vi "Lab Panel V6.00.vi"() -> ()   [LabVIEW 2017] (continued)
              tunnel: w5250 -> [w5255 w5288]
              tunnel: w5249 -> [w5254 w5287]
              tunnel: w5248 -> [w5253 _]
              tunnel: w5237 -> [_ w5286]
              tunnel: w5247 -> [_ w5285]
              tunnel: w5246 -> [_ w5284]
              tunnel: w5245 -> [_ w5283]
              tunnel: w5244 -> [_ w5282]
              tunnel: w5243 -> [_ w5281]
              tunnel: w5242 -> [_ w5280]
              tunnel: w5241 -> [_ w5279]
              tunnel: w5240 -> [_ w5278]
              tunnel: w5239 -> [_ w5277]
              tunnel: w5238 -> [_ w5276]
              tunnel: "TO (string):" -> [w5252 _]
              frame #0 {
                # "mail test"
                n2915 = case shown="True" w5253 {
                  tunnel: w5256 -> [_ w5260]
                  tunnel: w5252 -> [_ w5259]
                  tunnel: w5255 -> [_ w5258]
                  tunnel: w5254 -> [_ w5257]
                  frame False {
                  }
                  frame True {
                    n2916 = stacked-sequence {
                      seq-local: [_ _ w5270 _] -> [_ _ _ w5271]
                      tunnel: w5260 -> [w5263 _ _ w5275]
                      tunnel: w5259 -> [_ _ w5268 _]
                      tunnel: w5258 -> [_ _ w5266 _]
                      tunnel: w5257 -> [_ _ w5267 _]
                      frame #0 {
                        n2917 = Bundle(cluster=w5263, "TEST MAIL STATUS"="TEST START") -> (w5261:T8)  [unwired: 6 in]
                        n2918 = local write "MAIL SETTINGS"(w5261) -> ()
                      }
                      frame #1 {
                        n2919 = Wait (ms)(milliseconds to wait=500) -> ()  [unwired: 1 out]
                      }
                      frame #2 {
                        n2920 = call "sub vi - send mail v5.vi"("TO:"=w5268, "subject"="MAIL TEST FROM LAB PANEL", "from"=w5267, "out going server"=w5266, "message"="TEST MESSAGE") -> ("error out"=w5270:errorcluster)  [unwired: 10 in]
                      }
                      frame #3 {
                        n2921 = Bundle(cluster=w5275, "TEST MAIL"=FALSE, "TEST MAIL STATUS"="TEST END", "mail error"=w5271) -> (w5273:T8)  [unwired: 4 in]
                        n2922 = local write "MAIL SETTINGS"(w5273) -> ()
                      }
                    }
                  }
                }
              }
              frame #1 {
                # "mail report"
                n2923 = stacked-sequence {
                  seq-local: [_ w5333 _ _] -> [_ _ _ w5523]
                  seq-local: [_ _ w5436 _] -> [_ _ _ w5513]
                  seq-local: [w5300 _ _ _] -> [_ w5350 _ _]
                  seq-local: [w5299 _ _ _] -> [_ w5349 _ _]
                  seq-local: [w5297 _ _ _] -> [_ w5347 _ _]
                  seq-local: [w5298 _ _ _] -> [_ w5348 _ _]
                  seq-local: [w5296 _ _ _] -> [_ w5346 _ _]
                  seq-local: [w5295 _ _ _] -> [_ w5341 _ _]
                  seq-local: [w5294 _ _ _] -> [_ w5342 _ _]
                  seq-local: [w5293 _ _ _] -> [_ w5343 _ _]
                  seq-local: [w5292 _ _ _] -> [_ w5344 _ _]
                  seq-local: [w5291 _ _ _] -> [_ w5345 _ _]
                  tunnel: w5290 -> [_ _ _ w5524]
                  tunnel: w5289 -> [_ _ _ w5507]
                  tunnel: w5288 -> [_ _ _ w5521]
                  tunnel: w5287 -> [_ _ _ w5520]
                  tunnel: w5286 -> [w5331 _ _ w5515]
                  tunnel: w5285 -> [_ _ w5466 _]
                  tunnel: w5284 -> [_ _ w5463 _]
                  tunnel: w5283 -> [_ _ w5462 _]
                  tunnel: w5282 -> [_ _ w5461 _]
                  tunnel: w5281 -> [_ _ w5460 _]
                  tunnel: w5280 -> [_ _ w5459 _]
                  tunnel: w5279 -> [_ _ w5458 _]
                  tunnel: w5278 -> [_ _ w5457 _]
                  tunnel: w5277 -> [_ _ w5456 _]
                  tunnel: w5276 -> [_ _ w5455 _]
                  frame #0 {
                    n2924 = case shown="False" w5331 {
                      frame False {
                        n2925 = local write "mail control"("") -> ()
                      }
                      frame True {
                      }
                    }
                    n2926 = local read "SET LAB01-1"() -> (w5330:T6)
                    n2927 = local read "SET LAB01-2"() -> (w5329:T5)
                    n2928 = local read "SET LAB02-1"() -> (w5328:T5)
                    n2929 = local read "SET LAB02-2"() -> (w5327:T5)
                    n2930 = local read "SET LAB03-1"() -> (w5326:T5)
                    n2931 = local read "SET LAB04-1"() -> (w5324:T5)
                    n2932 = local read "SET LAB05-1"() -> (w5322:T5)
                    n2933 = local read "SET LAB03-2"() -> (w5325:T5)
                    n2934 = local read "SET LAB04-2"() -> (w5323:T5)
                    n2935 = local read "SET LAB05-2"() -> (w5321:T5)
                    n2936 = Unbundle(w5326) -> ("DESCRIPTION"=w5306:string)  [unwired: 4 out]
                    n2937 = Unbundle(w5325) -> ("DESCRIPTION"=w5305:string)  [unwired: 4 out]
                    n2938 = Unbundle(w5324) -> ("DESCRIPTION"=w5304:string)  [unwired: 4 out]
                    n2939 = Unbundle(w5321) -> ("DESCRIPTION"=w5301:string)  [unwired: 4 out]
                    n2940 = Unbundle(w5327) -> ("DESCRIPTION"=w5307:string)  [unwired: 4 out]
                    n2941 = Unbundle(w5323) -> ("DESCRIPTION"=w5303:string)  [unwired: 4 out]
                    n2942 = Unbundle(w5330) -> ("DESCRIPTION"=w5319:string)  [unwired: 4 out]
                    n2943 = Unbundle(w5328) -> ("DESCRIPTION"=w5308:string)  [unwired: 4 out]
                    n2944 = Unbundle(w5322) -> ("DESCRIPTION"=w5302:string)  [unwired: 4 out]
                    n2945 = Unbundle(w5329) -> ("DESCRIPTION"=w5309:string)  [unwired: 4 out]
                    n2946 = Concatenate Strings("[LAB05-2/", w5301) -> (w5291:string)
                    n2947 = Concatenate Strings("[LAB05-1/", w5302) -> (w5292:string)
                    n2948 = Concatenate Strings("[LAB04-2/", w5303) -> (w5293:string)
                    n2949 = Concatenate Strings("[LAB03-2/", w5305) -> (w5295:string)
                    n2950 = Concatenate Strings("[LAB04-1/", w5304) -> (w5294:string)
                    n2951 = Concatenate Strings("[LAB03-1/", w5306) -> (w5296:string)
                    n2952 = Concatenate Strings("[LAB01-2/", w5309) -> (w5299:string)
                    n2953 = Concatenate Strings("[LAB02-2/", w5307) -> (w5297:string)
                    n2954 = Concatenate Strings("[LAB01-1/", w5319) -> (w5300:string)
                    n2955 = Concatenate Strings("[LAB02-1/", w5308) -> (w5298:string)
                  }
                  frame #1 {
                    w5354 = "/"
                    w5355 = 2.0
                    n2956 = local read "DISP LAB01-1"() -> (w5435:T4)
                    n2957 = local read "DISP LAB01-2"() -> (w5434:T4)
                    n2958 = local read "DISP LAB02-1"() -> (w5433:T4)
                    n2959 = local read "DISP LAB03-2"() -> (w5430:T4)
                    n2960 = local read "DISP LAB02-2"() -> (w5432:T4)
                    n2961 = local read "DISP LAB03-1"() -> (w5431:T4)
                    n2962 = local read "DISP LAB04-2"() -> (w5428:T4)
                    n2963 = local read "DISP LAB04-1"() -> (w5429:T4)
                    n2964 = local read "DISP LAB05-1"() -> (w5427:T4)
                    n2965 = local read "DISP LAB05-2"() -> (w5426:T4)
                    n2966 = Unbundle By Name(w5435) -> ("CYCLE"=w5423:dbl, "MINS"=w5422:dbl, "STATUS"=w5419:string)
                    n2967 = Unbundle(w5434) -> ("CYCLE"=w5418:dbl, "MINS"=w5417:dbl, "STATUS"=w5414:string)
                    n2968 = Unbundle(w5433) -> ("CYCLE"=w5411:dbl, "MINS"=w5410:dbl, "STATUS"=w5409:string)
                    n2969 = Unbundle(w5430) -> ("CYCLE"=w5398:dbl, "MINS"=w5397:dbl, "STATUS"=w5394:string)
                    n2970 = Unbundle(w5431) -> ("CYCLE"=w5403:dbl, "MINS"=w5402:dbl, "STATUS"=w5399:string)
                    n2971 = Unbundle(w5432) -> ("CYCLE"=w5408:dbl, "MINS"=w5407:dbl, "STATUS"=w5404:string)
                    n2972 = Unbundle(w5429) -> ("CYCLE"=w5393:dbl, "MINS"=w5392:dbl, "STATUS"=w5389:string)
                    n2973 = Unbundle(w5428) -> ("CYCLE"=w5388:dbl, "MINS"=w5387:dbl, "STATUS"=w5384:string)
                    n2974 = Unbundle(w5427) -> ("CYCLE"=w5383:dbl, "MINS"=w5382:dbl, "STATUS"=w5379:string)
                    n2975 = Unbundle(w5426) -> ("CYCLE"=w5425:dbl, "MINS"=w5424:dbl, "STATUS"=w5376:string)
                    n2976 = Number To Decimal String(number=w5411) -> (decimal integer string=w5413:string)  [unwired: 1 in]
                    n2977 = Number To Decimal String(number=w5408) -> (decimal integer string=w5406:string)  [unwired: 1 in]
                    n2978 = Number To Decimal String(number=w5403) -> (decimal integer string=w5401:string)  [unwired: 1 in]
                    n2979 = Number To Decimal String(number=w5418) -> (decimal integer string=w5416:string)  [unwired: 1 in]
                    n2980 = Number To Decimal String(number=w5398) -> (decimal integer string=w5396:string)  [unwired: 1 in]
                    n2981 = Number To Decimal String(number=w5423) -> (decimal integer string=w5421:string)  [unwired: 1 in]
                    n2982 = Number To Decimal String(number=w5425) -> (decimal integer string=w5378:string)  [unwired: 1 in]
                    n2983 = Number To Decimal String(number=w5393) -> (decimal integer string=w5391:string)  [unwired: 1 in]
                    n2984 = Number To Decimal String(number=w5388) -> (decimal integer string=w5386:string)  [unwired: 1 in]
                    n2985 = Number To Decimal String(number=w5383) -> (decimal integer string=w5381:string)  [unwired: 1 in]
                    n2986 = Number To Fractional String(number=w5410, precision (6)=w5355) -> (F-format string=w5412:string)  [unwired: 2 in]
                    n2987 = Number To Fractional String(number=w5397, precision (6)=w5355) -> (F-format string=w5395:string)  [unwired: 2 in]
                    n2988 = Number To Fractional String(number=w5407, precision (6)=w5355) -> (F-format string=w5405:string)  [unwired: 2 in]
                    n2989 = Number To Fractional String(number=w5402, precision (6)=w5355) -> (F-format string=w5400:string)  [unwired: 2 in]
                    n2990 = Number To Fractional String(number=w5387, precision (6)=w5355) -> (F-format string=w5385:string)  [unwired: 2 in]
                    n2991 = Number To Fractional String(number=w5392, precision (6)=w5355) -> (F-format string=w5390:string)  [unwired: 2 in]
                    n2992 = Number To Fractional String(number=w5417, precision (6)=w5355) -> (F-format string=w5415:string)  [unwired: 2 in]
                    n2993 = Number To Fractional String(number=w5382, precision (6)=w5355) -> (F-format string=w5380:string)  [unwired: 2 in]
                    n2994 = Number To Fractional String(number=w5422, precision (6)=w5355) -> (F-format string=w5420:string)  [unwired: 2 in]
                    n2995 = Number To Fractional String(number=w5424, precision (6)=w5355) -> (F-format string=w5377:string)  [unwired: 2 in]
                    n2996 = Concatenate Strings(w5354, w5396, w5354, w5395, w5354, w5394) -> (w5370:string)
                    n2997 = Concatenate Strings(w5354, w5391, w5354, w5390, w5354, w5389) -> (w5369:string)
                    n2998 = Concatenate Strings(w5354, w5386, w5354, w5385, w5354, w5384) -> (w5368:string)
                    n2999 = Concatenate Strings(w5354, w5381, w5354, w5380, w5354, w5379) -> (w5367:string)
                    n3000 = Concatenate Strings(w5354, w5378, w5354, w5377, w5354, w5376) -> (w5366:string)
                    n3001 = Concatenate Strings(w5354, w5421, w5354, w5420, w5354, w5419) -> (w5375:string)
                    n3002 = Concatenate Strings(w5354, w5401, w5354, w5400, w5354, w5399) -> (w5371:string)
                    n3003 = Concatenate Strings(w5354, w5416, w5354, w5415, w5354, w5414) -> (w5374:string)
                    n3004 = Concatenate Strings(w5354, w5413, w5354, w5412, w5354, w5409) -> (w5373:string)
                    n3005 = Concatenate Strings(w5354, w5406, w5354, w5405, w5354, w5404) -> (w5372:string)
                    n3006 = Concatenate Strings("]", "\r") -> (w5351:string)
                    n3007 = Concatenate Strings(w5346, w5371, w5351) -> (w5361:string)
                    n3008 = Concatenate Strings(w5348, w5373, w5351) -> (w5363:string)
                    n3009 = Concatenate Strings(w5347, w5372, w5351) -> (w5362:string)
                    n3010 = Concatenate Strings(w5343, w5368, w5351) -> (w5358:string)
                    n3011 = Concatenate Strings(w5344, w5367, w5351) -> (w5359:string)
                    n3012 = Concatenate Strings(w5342, w5369, w5351) -> (w5357:string)
                    n3013 = Concatenate Strings(w5341, w5370, w5351) -> (w5356:string)
                    n3014 = Concatenate Strings(w5345, w5366, w5351) -> (w5360:string)
                    n3015 = Concatenate Strings(w5349, w5374, w5351) -> (w5364:string)
                    n3016 = Concatenate Strings(w5350, w5375, w5351) -> (w5365:string)
                    n3017 = Concatenate Strings(w5365, w5364, w5363, w5362, w5361, w5356, w5357, w5358, w5359, w5360) -> (w5334:string)
                    n3018 = Concatenate Strings("[PANEL/", "DESC/", "CYCLES/", "MINS/", "STATUS]", "\r", w5334) -> (w5333:string)
                    "MAIL REPORT" <- w5333
                    n3019 = global write "Global display 3.vi" "log all"(w5333) -> ()
                  }
                  frame #2 {
                    w5464 = "END"
                    n3020 = local read "mail control"() -> (w5465:string)
                    n3021 = case shown="False" w5460 {
                      tunnel: w5465 -> [w5489 _]
                      tunnel: w5464 -> [w5488 _]
                      tunnel: [w5487 FALSE] -> w5450
                      frame False {
                        n3022 = Equal?(x=w5489, y=w5488) -> (x = y?=w5487:bool)
                      }
                      frame True {
                      }
                    }
                    n3023 = case shown="False" w5466 {
                      tunnel: w5465 -> [w5505 _]
                      tunnel: w5464 -> [w5504 _]
                      tunnel: [w5503 FALSE] -> w5454
                      frame False {
                        n3024 = Equal?(x=w5505, y=w5504) -> (x = y?=w5503:bool)
                      }
                      frame True {
                      }
                    }
                    n3025 = case shown="False" w5463 {
                      tunnel: w5465 -> [w5501 _]
                      tunnel: w5464 -> [w5500 _]
                      tunnel: [w5499 FALSE] -> w5453
                      frame False {
                        n3026 = Equal?(x=w5501, y=w5500) -> (x = y?=w5499:bool)
                      }
                      frame True {
                      }
                    }
                    n3027 = case shown="False" w5461 {
                      tunnel: w5465 -> [w5493 _]
                      tunnel: w5464 -> [w5492 _]
                      tunnel: [w5491 FALSE] -> w5451
                      frame False {
                        n3028 = Equal?(x=w5493, y=w5492) -> (x = y?=w5491:bool)
                      }
                      frame True {
                      }
                    }
                    n3029 = case shown="False" w5462 {
                      tunnel: w5465 -> [w5497 _]
                      tunnel: w5464 -> [w5496 _]
                      tunnel: [w5495 FALSE] -> w5452
                      frame False {
                        n3030 = Equal?(x=w5497, y=w5496) -> (x = y?=w5495:bool)
                      }
                      frame True {
                      }
                    }
                    n3031 = Or(x=w5452, y=w5451) -> (x .or. y?=w5443:bool)
                    n3032 = Or(x=w5454, y=w5453) -> (x .or. y?=w5444:bool)
                    n3033 = Or(x=w5444, y=w5443) -> (x .or. y?=w5439:bool)
                    n3034 = case shown="False" w5456 {
                      tunnel: w5465 -> [w5473 _]
                      tunnel: w5464 -> [w5472 _]
                      tunnel: [w5471 FALSE] -> w5445
                      frame False {
                        n3035 = Equal?(x=w5473, y=w5472) -> (x = y?=w5471:bool)
                      }
                      frame True {
                      }
                    }
                    n3036 = case shown="False" w5455 {
                      tunnel: w5465 -> [w5469 _]
                      tunnel: w5464 -> [w5468 _]
                      tunnel: [w5467 FALSE] -> w5449
                      frame False {
                        n3037 = Equal?(x=w5469, y=w5468) -> (x = y?=w5467:bool)
                      }
                      frame True {
                      }
                    }
                    n3038 = case shown="False" w5457 {
                      tunnel: w5465 -> [w5477 _]
                      tunnel: w5464 -> [w5476 _]
                      tunnel: [w5475 FALSE] -> w5446
                      frame False {
                        n3039 = Equal?(x=w5477, y=w5476) -> (x = y?=w5475:bool)
                      }
                      frame True {
                      }
                    }
                    n3040 = case shown="False" w5459 {
                      tunnel: w5465 -> [w5485 _]
                      tunnel: w5464 -> [w5484 _]
                      tunnel: [w5483 FALSE] -> w5448
                      frame False {
                        n3041 = Equal?(x=w5485, y=w5484) -> (x = y?=w5483:bool)
                      }
                      frame True {
                      }
                    }
                    n3042 = case shown="False" w5458 {
                      tunnel: w5465 -> [w5481 _]
                      tunnel: w5464 -> [w5480 _]
                      tunnel: [w5479 FALSE] -> w5447
                      frame False {
                        n3043 = Equal?(x=w5481, y=w5480) -> (x = y?=w5479:bool)
                      }
                      frame True {
                      }
                    }
                    n3044 = Or(x=w5448, y=w5447) -> (x .or. y?=w5442:bool)
                    n3045 = Or(x=w5446, y=w5445) -> (x .or. y?=w5441:bool)
                    n3046 = Or(x=w5449, y=w5450) -> (x .or. y?=w5437:bool)
                    n3047 = Or(x=w5442, y=w5441) -> (x .or. y?=w5440:bool)
                    n3048 = Or(x=w5439, y=w5440) -> (x .or. y?=w5438:bool)
                    n3049 = Or(x=w5438, y=w5437) -> (x .or. y?=w5436:bool)
                  }
                  frame #3 {
                    n3050 = local read "on loops"() -> (w5519:dbl)
                    n3051 = local read "jig cycle"() -> (w5516:dbl)
                    n3052 = local read "Send Mail Now"() -> (w5510:bool)
                    n3053 = Add(x=w5519, y=5.0) -> (x+y=w5517:dbl)
                    n3054 = Equal?(x=w5516, y=w5517) -> (x = y?=w5511:bool)
                    n3055 = And(x=w5511, y=w5510) -> (x .and. y?=w5509:bool)
                    n3056 = And(x=w5515, y=w5511) -> (x .and. y?=w5514:bool)
                    n3057 = And(x=w5514, y=w5513) -> (x .and. y?=w5512:bool)
                    n3058 = Or(x=w5512, y=w5509) -> (x .or. y?=w5508:bool)
                    n3059 = case shown="True" w5508 {
                      tunnel: w5524 -> [_ w5530]
                      tunnel: w5523 -> [_ w5529]
                      tunnel: "Lab Panel Test Status" -> [_ w5528]
                      tunnel: w5521 -> [_ w5527]
                      tunnel: w5520 -> [_ w5526]
                      tunnel: w5507 -> [_ w5525]
                      frame False {
                      }
                      frame True {
                        n3060 = stacked-sequence {
                          tunnel: w5530 -> [w5539 _]
                          tunnel: w5529 -> [w5538 _]
                          tunnel: w5528 -> [w5537 _]
                          tunnel: w5527 -> [w5536 _]
                          tunnel: w5526 -> [w5535 _]
                          tunnel: w5525 -> [w5534 _]
                          frame #0 {
                            n3061 = call "sub vi - send mail v5.vi"("TO:"=w5539, "subject"=w5537, "Info"="Test station status report", "from"=w5535, "out going server"=w5536, "message"=w5538) -> ("error out"=w5533:errorcluster)  [unwired: 9 in]
                            n3062 = Bundle(cluster=w5534, "mail error"=w5533) -> (w5532:T8)  [unwired: 6 in]
                            n3063 = local write "MAIL SETTINGS"(w5532) -> ()
                          }
                          frame #1 {
                            n3064 = local write "mail control"("") -> ()
                            n3065 = local write "Send Mail Now"(FALSE) -> ()
                          }
                        }
                      }
                    }
                  }
                }
              }
            }
          }
          frame #20 {
            # "save jig cycle values once all run switches are off"
            n3066 = stacked-sequence {
              tunnel: w5551 -> [_ w5580]
              tunnel: w5550 -> [_ w5579]
              tunnel: w5549 -> [_ w5578]
              tunnel: w5548 -> [_ w5577]
              tunnel: w5547 -> [_ w5576]
              tunnel: w5546 -> [_ w5575]
              tunnel: w5545 -> [_ w5574]
              tunnel: w5544 -> [_ w5573]
              tunnel: w5543 -> [_ w5572]
              tunnel: w5542 -> [_ w5571]
              frame #0 {
              }
              frame #1 {
                n3067 = Not(x=w5571) -> (.not. x?=w5554:bool)
                n3068 = Not(x=w5579) -> (.not. x?=w5569:bool)
                n3069 = Not(x=w5576) -> (.not. x?=w5564:bool)
                n3070 = Not(x=w5574) -> (.not. x?=w5560:bool)
                n3071 = Not(x=w5572) -> (.not. x?=w5556:bool)
                n3072 = Not(x=w5580) -> (.not. x?=w5570:bool)
                n3073 = Not(x=w5578) -> (.not. x?=w5568:bool)
                n3074 = Not(x=w5575) -> (.not. x?=w5562:bool)
                n3075 = Not(x=w5577) -> (.not. x?=w5566:bool)
                n3076 = Not(x=w5573) -> (.not. x?=w5558:bool)
                n3077 = local read "Save JC"() -> (w5582:bool)
                n3078 = And(x=w5570, y=w5569) -> (x .and. y?=w5567:bool)
                n3079 = And(x=w5567, y=w5568) -> (x .and. y?=w5565:bool)
                n3080 = And(x=w5565, y=w5566) -> (x .and. y?=w5563:bool)
                n3081 = And(x=w5563, y=w5564) -> (x .and. y?=w5561:bool)
                n3082 = And(x=w5561, y=w5562) -> (x .and. y?=w5559:bool)
                n3083 = And(x=w5559, y=w5560) -> (x .and. y?=w5557:bool)
                n3084 = And(x=w5557, y=w5558) -> (x .and. y?=w5555:bool)
                n3085 = And(x=w5555, y=w5556) -> (x .and. y?=w5553:bool)
                n3086 = And(x=w5553, y=w5554) -> (x .and. y?=w5552:bool)
                n3087 = And(x=w5552, y=w5582) -> (x .and. y?=w5581:bool)
                n3088 = case shown="True" w5581 {
                  tunnel: w5552 -> [w5583 _]
                  frame False {
                    n3089 = case shown="False" w5583 {
                      frame False {
                        n3090 = local write "Save JC"(TRUE) -> ()
                      }
                      frame True {
                      }
                    }
                  }
                  frame True {
                    n3091 = stacked-sequence {
                      frame #0 {
                        n3092 = String To Path(string="c:\\crabtree\\Jig Cycles\\") -> (path=w5595:path)
                        n3093 = Build Path(base path=w5595, name or relative path="jigcycles.bin") -> (appended path=w5593:path)
                        n3094 = Create Folder(path (use dialog)=w5595) -> (error out=w5597:errorcluster)  [unwired: 2 in, 2 out]
                        n3095 = local read "JIG RELAY CYCLES"() -> (w5587:T9)
                        n3096 = call <vilib>:"Clear Errors.vi"("error in (no error)"=w5597) -> ()  [unwired: 5 in, 2 out]
                        n3097 = local write "Save JC"(FALSE) -> ()
                        n3098 = Open/Create/Replace File(file path (use dialog)=w5593, operation (0:open)=T18."replace or create") -> (refnum out=w5591:refnum<file>, error out=w5592:errorcluster)  [unwired: 4 in, 1 out]
                        n3099 = Write to Binary File(file (use dialog)=w5591, data=w5587, error in=w5592) -> (refnum out=w5590:refnum<file>, error out=w5589:errorcluster)  [unwired: 3 in, 1 out]
                        n3100 = Close File(refnum=w5590, error in=w5589) -> (error out=w5588:errorcluster)  [unwired: 1 out]
                        n3101 = local write "data file error"(w5588) -> ()
                      }
                      frame #1 {
                        n3102 = local read "JIG RELAY CYCLES"() -> (w5620:T9)
                        n3103 = Unbundle By Name(w5620) -> ("LAB01-1"=w5615:dbl, "LAB01-2"=w5614:dbl, "LAB02-1"=w5612:dbl, "LAB02-2"=w5611:dbl, "LAB03-1"=w5609:dbl, "LAB03-2"=w5606:dbl, "LAB04-1"=w5605:dbl, "LAB04-2"=w5603:dbl, "LAB05-1"=w5601:dbl, "LAB05-2"=w5599:dbl)
                        n3104 = stacked-sequence {
                          tunnel: w5615 -> [w5623 _ _ _ _ _ _ _ _ _]
                          tunnel: 1000000 -> [w5626 w5636 w5646 w5656 w5666 w5676 w5686 w5696 w5706 w5716]
                          tunnel: [w5624 _ _ _ _ _ _ _ _ _] -> w5618
                          tunnel: "TEST STATION HAS REACHED 1 MILLION CYCLES, REPLACE  CONTROL RELAYS" -> [w5622 w5634 w5644 w5654 w5664 w5674 w5684 w5694 w5704 w5714]
                          tunnel: [_ w5633 _ _ _ _ _ _ _ _] -> w5616
                          tunnel: w5614 -> [_ w5632 _ _ _ _ _ _ _ _]
                          tunnel: [_ _ w5643 _ _ _ _ _ _ _] -> w5613
                          tunnel: w5612 -> [_ _ w5642 _ _ _ _ _ _ _]
                          tunnel: w5611 -> [_ _ _ w5653 _ _ _ _ _ _]
                          tunnel: [_ _ _ w5652 _ _ _ _ _ _] -> w5610
                          tunnel: w5609 -> [_ _ _ _ w5663 _ _ _ _ _]
                          tunnel: [_ _ _ _ w5662 _ _ _ _ _] -> w5608
                          tunnel: [_ _ _ _ _ w5673 _ _ _ _] -> w5607
                          tunnel: w5606 -> [_ _ _ _ _ w5672 _ _ _ _]
                          tunnel: w5605 -> [_ _ _ _ _ _ w5683 _ _ _]
                          tunnel: [_ _ _ _ _ _ w5682 _ _ _] -> w5604
                          tunnel: w5603 -> [_ _ _ _ _ _ _ w5693 _ _]
                          tunnel: [_ _ _ _ _ _ _ w5692 _ _] -> w5602
                          tunnel: w5601 -> [_ _ _ _ _ _ _ _ w5703 _]
                          tunnel: [_ _ _ _ _ _ _ _ w5702 _] -> w5600
                          tunnel: w5599 -> [_ _ _ _ _ _ _ _ _ w5713]
                          tunnel: [_ _ _ _ _ _ _ _ _ w5712] -> w5598
                          frame #0 {
                            n3105 = Greater?(x=w5623, y=w5626) -> (0:w5625:bool)
                            n3106 = case shown="True" w5625 {
                              tunnel: [w5627 0] -> w5624
                              tunnel: w5623 -> [w5627 _]
                              tunnel: w5622 -> [_ w5628]
                              frame False {
                              }
                              frame True {
                                n3107 = Concatenate Strings("LA01-1 ", w5628) -> (w5631:string)
                                n3108 = One Button Dialog(message=w5631) -> ()  [unwired: 1 in, 1 out]
                              }
                            }
                          }
                          frame #1 {
                            n3109 = Greater?(x=w5632, y=w5636) -> (0:w5635:bool)
                            n3110 = case shown="True" w5635 {
                              tunnel: [w5637 0] -> w5633
                              tunnel: w5632 -> [w5637 _]
                              tunnel: w5634 -> [_ w5638]
                              frame False {
                              }
                              frame True {
                                n3111 = Concatenate Strings("LA01-2 ", w5638) -> (w5641:string)
                                n3112 = One Button Dialog(message=w5641) -> ()  [unwired: 1 in, 1 out]
                              }
                            }
                          }
                          frame #2 {
                            n3113 = Greater?(x=w5642, y=w5646) -> (0:w5645:bool)
                            n3114 = case shown="True" w5645 {
                              tunnel: [w5647 0] -> w5643
                              tunnel: w5642 -> [w5647 _]
                              tunnel: w5644 -> [_ w5648]
                              frame False {
                              }
                              frame True {
                                n3115 = Concatenate Strings("LA02-1 ", w5648) -> (w5651:string)
                                n3116 = One Button Dialog(message=w5651) -> ()  [unwired: 1 in, 1 out]
                              }
                            }
                          }
                          frame #3 {
                            n3117 = Greater?(x=w5653, y=w5656) -> (0:w5655:bool)
                            n3118 = case shown="True" w5655 {
                              tunnel: [w5657 0] -> w5652
                              tunnel: w5653 -> [w5657 _]
                              tunnel: w5654 -> [_ w5658]
                              frame False {
                              }
                              frame True {
                                n3119 = Concatenate Strings("LA02-2 ", w5658) -> (w5661:string)
                                n3120 = One Button Dialog(message=w5661) -> ()  [unwired: 1 in, 1 out]
                              }
                            }
                          }
                          frame #4 {
                            n3121 = Greater?(x=w5663, y=w5666) -> (0:w5665:bool)
                            n3122 = case shown="True" w5665 {
                              tunnel: [w5667 0] -> w5662
                              tunnel: w5663 -> [w5667 _]
                              tunnel: w5664 -> [_ w5668]
                              frame False {
                              }
                              frame True {
                                n3123 = Concatenate Strings("LA03-1 ", w5668) -> (w5671:string)
                                n3124 = One Button Dialog(message=w5671) -> ()  [unwired: 1 in, 1 out]
                              }
                            }
                          }
                          frame #5 {
                            n3125 = Greater?(x=w5672, y=w5676) -> (0:w5675:bool)
                            n3126 = case shown="True" w5675 {
                              tunnel: [w5677 0] -> w5673
                              tunnel: w5672 -> [w5677 _]
                              tunnel: w5674 -> [_ w5678]
                              frame False {
                              }
                              frame True {
                                n3127 = Concatenate Strings("LA03-2 ", w5678) -> (w5681:string)
                                n3128 = One Button Dialog(message=w5681) -> ()  [unwired: 1 in, 1 out]
                              }
                            }
                          }
                          frame #6 {
                            n3129 = Greater?(x=w5683, y=w5686) -> (0:w5685:bool)
                            n3130 = case shown="True" w5685 {
                              tunnel: [w5687 0] -> w5682
                              tunnel: w5683 -> [w5687 _]
                              tunnel: w5684 -> [_ w5688]
                              frame False {
                              }
                              frame True {
                                n3131 = Concatenate Strings("LA04-1 ", w5688) -> (w5691:string)
                                n3132 = One Button Dialog(message=w5691) -> ()  [unwired: 1 in, 1 out]
                              }
                            }
                          }
                          frame #7 {
                            n3133 = Greater?(x=w5693, y=w5696) -> (0:w5695:bool)
                            n3134 = case shown="True" w5695 {
                              tunnel: [w5697 0] -> w5692
                              tunnel: w5693 -> [w5697 _]
                              tunnel: w5694 -> [_ w5698]
                              frame False {
                              }
                              frame True {
                                n3135 = Concatenate Strings("LA04-2 ", w5698) -> (w5701:string)
                                n3136 = One Button Dialog(message=w5701) -> ()  [unwired: 1 in, 1 out]
                              }
                            }
                          }
                          frame #8 {
                            n3137 = Greater?(x=w5703, y=w5706) -> (0:w5705:bool)
                            n3138 = case shown="True" w5705 {
                              tunnel: [w5707 0] -> w5702
                              tunnel: w5703 -> [w5707 _]
                              tunnel: w5704 -> [_ w5708]
                              frame False {
                              }
                              frame True {
                                n3139 = Concatenate Strings("LA05-1 ", w5708) -> (w5711:string)
                                n3140 = One Button Dialog(message=w5711) -> ()  [unwired: 1 in, 1 out]
                              }
                            }
                          }
                          frame #9 {
                            n3141 = Greater?(x=w5713, y=w5716) -> (0:w5715:bool)
                            n3142 = case shown="True" w5715 {
                              tunnel: [w5717 0] -> w5712
                              tunnel: w5713 -> [w5717 _]
                              tunnel: w5714 -> [_ w5718]
                              frame False {
                              }
                              frame True {
                                n3143 = Concatenate Strings("LA05-2 ", w5718) -> (w5721:string)
                                n3144 = One Button Dialog(message=w5721) -> ()  [unwired: 1 in, 1 out]
                              }
                            }
                          }
                        }
                        n3145 = Bundle By Name(cluster=w5620, "LAB01-1"=w5618, "LAB01-2"=w5616, "LAB02-1"=w5613, "LAB02-2"=w5610, "LAB03-1"=w5608, "LAB03-2"=w5607, "LAB04-1"=w5604, "LAB04-2"=w5602, "LAB05-1"=w5600, "LAB05-2"=w5598) -> (w5619:T9)
                        n3146 = local write "JIG RELAY CYCLES"(w5619) -> ()
                      }
                    }
                  }
                }
              }
            }
          }
          frame #21 {
            # "get temperature values"
            n3147 = local read "Simulate"() -> (w5734:bool)
            n3148 = local read "Temp Test Cal"() -> (w5731:dbl)
            n3149 = stacked-sequence {
              seq-local: [_ w5741 _] -> [_ _ w5786]
              tunnel: w5734 -> [_ _ w5799]
              tunnel: T15 {"1  (A) cal"=1.0, "1 (V) cal"=1.0, "1 (PF) cal"=1.0, "1 (TL) cal"=1.0, "1 (TN) cal"=1.0, "2 (A) cal"=1.0, "2 (V) cal"=1.0, "2 (PF) cal"=1.0, "2 (TL) cal"=1.0, "2 (TN) cal"=1.0} ("CAL LAB01") -> [_ _ w5798]
              tunnel: w5732 -> [_ _ w5797]
              tunnel: w5731 -> [_ _ w5796]
              tunnel: w5730 -> [_ _ w5795]
              tunnel: w5729 -> [_ _ w5794]
              tunnel: w5728 -> [_ _ w5793]
              tunnel: w5727 -> [_ _ w5792]
              tunnel: w5726 -> [_ _ w5791]
              tunnel: w5725 -> [_ _ w5790]
              tunnel: w5724 -> [_ _ w5789]
              tunnel: w5723 -> [_ _ w5788]
              tunnel: w5722 -> [_ _ w5787]
              frame #0 {
                n3150 = case shown="True" "Open Com Port" {
                  frame False {
                  }
                  frame True {
                    n3151 = local read "Select COM port"() -> (w5739:refnum<visa-resource-name>)
                    n3152 = call "sub vi-open serial port v1.vi"("Select COM port"=w5739) -> ("Error"=w5738:bool, "LOOPS"=w5737:i32, "VISA Com out"=w5736:refnum<visa-resource-name>)  [unwired: 12 in]
                    n3153 = local write "Com setup loops"(w5737) -> ()
                    n3154 = local write "Com Port Status"(w5738) -> ()
                    n3155 = local write "VISA Com out"(w5736) -> ()
                    n3156 = global write "Global 1.vi" "COM port"(w5736) -> ()
                  }
                }
              }
              frame #1 {
                # "only get temperature from initial valid temperature circuits, circuits detected at startup time"
                n3157 = local read "VISA Com out"() -> (w5749:refnum<visa-resource-name>)
                n3158 = global write "Global 1.vi" "COM port"(w5749) -> ()
                n3159 = local read "Temp read loop"() -> (w5746:dbl)
                n3160 = global write "Global 1.vi" "tmp dly lps"("Temp Delay Lps") -> ()
                n3161 = global write "Global 1.vi" "dly value"("Temp Value") -> ()
                n3162 = local read "jig cycle"() -> (w5750:dbl)
                n3163 = local read "on loops"() -> (w5752:dbl)
                n3164 = Equal?(x=w5746, y=1) -> (x = y?=w5743:bool)
                n3165 = Add(x=w5752, y=6) -> (x+y=w5753:dbl)
                n3166 = Equal?(x=w5750, y=w5753) -> (x = y?=w5744:bool)
                n3167 = And(x=w5744, y=w5743) -> (x .and. y?=w5742:bool)
                n3168 = Or(x=w5742, y="Read Temp") -> (x .or. y?=w5741:bool)
                n3169 = case shown="True" w5741 {
                  frame False {
                  }
                  frame True {
                    n3170 = local read "Simulate"() -> (w5755:bool)
                    n3171 = local write "TEMP"(TRUE) -> ()
                    n3172 = local write "Read Temp"(FALSE) -> ()
                    n3173 = stacked-sequence {
                      tunnel: 1.0 -> [_ _ _ _ w5785]
                      tunnel: w5755 -> [_ _ _ _ w5784]
                      frame #0 {
                        # "only switch relay on to reset temp circuits if busy testing"
                        n3174 = disable-structure shown="Disabled" {
                          frame Disabled {
                            n3175 = local read "Any Test Running"() -> ()  [unwired: 1 out]
                          }
                          frame Enabled {
                          }
                        }
                        n3176 = local read "USB OUT 0"() -> (w5759:bool[])
                        n3177 = local read "USB OUT 2"() -> (w5761:bool[])
                        n3178 = local read "USB OUT 1"() -> (w5760:bool[])
                        n3179 = Insert Into Array(array=w5761, index=7, new element=TRUE) -> (w5762:bool[])
                        n3180 = call "sub vi - Drive Relays All v6.vi"("Array #2"=w5762, "Array #1"=w5760, "Array #0"=w5759) -> ()  [unwired: 8 in, 1 out]
                      }
                      frame #1 {
                        # "time delay"
                        n3181 = Wait (ms)(milliseconds to wait=500) -> ()  [unwired: 1 out]
                      }
                      frame #2 {
                        # "switch relay off"
                        n3182 = local read "USB OUT 0"() -> (w5765:bool[])
                        n3183 = local read "USB OUT 2"() -> (w5767:bool[])
                        n3184 = local read "USB OUT 1"() -> (w5766:bool[])
                        n3185 = Insert Into Array(array=w5767, index=7, new element=FALSE) -> (w5768:bool[])
                        n3186 = call "sub vi - Drive Relays All v6.vi"("Array #2"=w5768, "Array #1"=w5766, "Array #0"=w5765) -> ()  [unwired: 8 in, 1 out]
                      }
                      frame #3 {
                        # "time delay"
                        n3187 = Wait (ms)(milliseconds to wait=300) -> ()  [unwired: 1 out]
                      }
                      frame #4 {
                        # "read all valid temp circuits"
                        n3188 = local read "LAB01-TP"() -> (w5777:bool)
                        n3189 = local read "LAB03-TP"() -> (w5775:bool)
                        n3190 = local read "LAB02-TP"() -> (w5776:bool)
                        n3191 = local read "LAB04-TP"() -> (w5774:bool)
                        n3192 = local read "LAB05-TP"() -> (w5778:bool)
                        n3193 = call "sub vi - GET ALL TEMP v7.vi"("LA01-EN"=w5777, "simulate"=w5784, "LA02-EN"=w5776, "LA03-EN"=w5775, "LA04-EN"=w5774, "LA05-EN"=w5778, "Gen Cal Value"=w5785) -> ("LOOP TIME"=→"Read Time":dbl, "LA01 TEMP"=w5783:T27, "LA02 TEMP"=w5782:T27, "LA03 TEMP"=w5781:T27, "LA04 TEMP"=w5780:T27, "error"=→"Error Temp":bool, "LA05 TEMP"=w5779:T27)  [unwired: 1 in, 1 out]
                        n3194 = local write "LAB01 TEMP"(w5783) -> ()
                        n3195 = local write "LAB02 TEMP"(w5782) -> ()
                        n3196 = local write "LAB03 TEMP"(w5781) -> ()
                        n3197 = local write "LAB04 TEMP"(w5780) -> ()
                        n3198 = local write "LAB05 TEMP"(w5779) -> ()
                      }
                    }
                  }
                }
              }
              frame #2 {
                n3199 = case shown="True" w5786 {
                  tunnel: w5799 -> [_ w5812]
                  tunnel: w5798 -> [_ w5811]
                  tunnel: w5797 -> [_ w5810]
                  tunnel: w5796 -> [_ w5809]
                  tunnel: w5795 -> [_ w5808]
                  tunnel: w5794 -> [_ w5807]
                  tunnel: w5793 -> [_ w5806]
                  tunnel: w5792 -> [_ w5805]
                  tunnel: w5791 -> [_ w5804]
                  tunnel: w5790 -> [_ w5803]
                  tunnel: w5789 -> [_ w5802]
                  tunnel: w5788 -> [_ w5801]
                  tunnel: w5787 -> [_ w5800]
                  frame False {
                  }
                  frame True {
                    n3200 = stacked-sequence {
                      tunnel: w5812 -> [_ w5825 w5870 w5915 w5960 w6005 _]
                      tunnel: w5811 -> [_ w5824 w5869 w5914 w5959 w6004 _]
                      tunnel: w5810 -> [_ w5814 _ _ _ _ _]
                      tunnel: w5809 -> [_ w5819 w5868 w5913 w5958 w6003 _]
                      tunnel: w5808 -> [_ w5813 _ _ _ _ _]
                      tunnel: w5807 -> [_ _ w5859 _ _ _ _]
                      tunnel: w5806 -> [_ _ w5858 _ _ _ _]
                      tunnel: w5805 -> [_ _ _ w5904 _ _ _]
                      tunnel: w5804 -> [_ _ _ w5903 _ _ _]
                      tunnel: w5803 -> [_ _ _ _ w5949 _ _]
                      tunnel: w5802 -> [_ _ _ _ w5948 _ _]
                      tunnel: w5801 -> [_ _ _ _ _ w5994 _]
                      tunnel: w5800 -> [_ _ _ _ _ w5993 _]
                      frame #0 {
                      }
                      frame #1 {
                        n3201 = case shown="False" w5825 {
                          tunnel: [w5856 w5857] -> w5841
                          tunnel: w5824 -> [_ w5857]
                          frame False {
                            n3202 = local read "CAL LAB01"() -> (w5856:T15)
                          }
                          frame True {
                          }
                        }
                        n3203 = local read "TEMP LA01"() -> (w5832:T10)
                        n3204 = local read "LAB01 TEMP"() -> (w5831:T13)
                        n3205 = call "sub vi - temperature delay v4.vi"("2-run"=w5813, "1-run"=w5814, "temp values IN"=w5832, "temp signals"=w5831) -> ("T2-N"=w5827:dbl, "T2-L"=w5828:dbl, "T1-N"=w5829:dbl, "T1-L"=w5830:dbl, "temp values OUT"=w5826:T47)  [unwired: 3 in]
                        n3206 = Unbundle By Name(w5841) -> ("1 (TL) cal"=w5836:dbl, "1 (TN) cal"=w5835:dbl, "2 (TL) cal"=w5834:dbl, "2 (TN) cal"=w5833:dbl)  [unwired: 6 out]
                        n3207 = local write "TEMP LA01"(w5826) -> ()
                        n3208 = Multiply(x=w5830, y=w5836) -> (x*y=w5823:dbl)
                        n3209 = Multiply(x=w5829, y=w5835) -> (x*y=w5821:dbl)
                        n3210 = Multiply(x=w5828, y=w5834) -> (x*y=w5818:dbl)
                        n3211 = Multiply(x=w5827, y=w5833) -> (x*y=w5817:dbl)
                        n3212 = case shown="True" w5814 {
                          tunnel: w5823 -> [w5850 w5855]
                          tunnel: w5819 -> [_ w5853]
                          tunnel: [w5850 w5854] -> w5822
                          tunnel: w5821 -> [w5849 w5852]
                          tunnel: [w5849 w5851] -> w5820
                          frame False {
                          }
                          frame True {
                            n3213 = Multiply(x=w5853, y=w5852) -> (x*y=w5851:dbl)
                            n3214 = Multiply(x=w5853, y=w5855) -> (x*y=w5854:dbl)
                          }
                        }
                        n3215 = case shown="True" w5813 {
                          tunnel: w5818 -> [w5843 w5848]
                          tunnel: w5819 -> [_ w5846]
                          tunnel: [w5843 w5847] -> w5816
                          tunnel: w5817 -> [w5842 w5845]
                          tunnel: [w5842 w5844] -> w5815
                          frame False {
                          }
                          frame True {
                            n3216 = Multiply(x=w5846, y=w5845) -> (x*y=w5844:dbl)
                            n3217 = Multiply(x=w5846, y=w5848) -> (x*y=w5847:dbl)
                          }
                        }
                        n3218 = local read "SIG LAB01-2"() -> (w5838:T2)
                        n3219 = local read "SIG LAB01-1"() -> (w5840:T2)
                        n3220 = Bundle By Name(cluster=w5840, "Tmp Live"=w5822, "Tmp Neut"=w5820) -> (w5839:T2)
                        n3221 = Bundle By Name(cluster=w5838, "Tmp Live"=w5816, "Tmp Neut"=w5815) -> (w5837:T2)
                        n3222 = local write "SIG LAB01-1"(w5839) -> ()
                        n3223 = local write "SIG LAB01-2"(w5837) -> ()
                      }
                      frame #2 {
                        n3224 = case shown="True" w5870 {
                          tunnel: [w5901 w5902] -> w5886
                          tunnel: w5869 -> [_ w5902]
                          frame False {
                            n3225 = local read "CAL LAB02"() -> (w5901:T16)
                          }
                          frame True {
                          }
                        }
                        n3226 = local read "LAB02 TEMP"() -> (w5877:T13)
                        n3227 = local read "TEMP LA02"() -> (w5876:T10)
                        n3228 = call "sub vi - temperature delay v4.vi"("2-run"=w5858, "1-run"=w5859, "temp values IN"=w5876, "temp signals"=w5877) -> ("T2-N"=w5871:dbl, "T2-L"=w5872:dbl, "T1-N"=w5873:dbl, "T1-L"=w5874:dbl, "temp values OUT"=w5875:T47)  [unwired: 3 in]
                        n3229 = Unbundle By Name(w5886) -> ("1 (TL) cal"=w5881:dbl, "1 (TN) cal"=w5880:dbl, "2 (TL) cal"=w5879:dbl, "2 (TN) cal"=w5878:dbl)  [unwired: 6 out]
                        n3230 = local write "TEMP LA02"(w5875) -> ()
                        n3231 = Multiply(x=w5874, y=w5881) -> (x*y=w5867:dbl)
                        n3232 = Multiply(x=w5873, y=w5880) -> (x*y=w5866:dbl)
                        n3233 = Multiply(x=w5872, y=w5879) -> (x*y=w5863:dbl)
                        n3234 = Multiply(x=w5871, y=w5878) -> (x*y=w5862:dbl)
                        n3235 = case shown="True" w5859 {
                          tunnel: w5867 -> [w5895 w5900]
                          tunnel: w5868 -> [_ w5898]
                          tunnel: [w5895 w5899] -> w5865
                          tunnel: w5866 -> [w5894 w5897]
                          tunnel: [w5894 w5896] -> w5864
                          frame False {
                          }
                          frame True {
                            n3236 = Multiply(x=w5898, y=w5897) -> (x*y=w5896:dbl)
                            n3237 = Multiply(x=w5898, y=w5900) -> (x*y=w5899:dbl)
                          }
                        }
                        n3238 = case shown="True" w5858 {
                          tunnel: w5863 -> [w5888 w5893]
                          tunnel: w5868 -> [_ w5891]
                          tunnel: [w5888 w5892] -> w5861
                          tunnel: w5862 -> [w5887 w5890]
                          tunnel: [w5887 w5889] -> w5860
                          frame False {
                          }
                          frame True {
                            n3239 = Multiply(x=w5891, y=w5890) -> (x*y=w5889:dbl)
                            n3240 = Multiply(x=w5891, y=w5893) -> (x*y=w5892:dbl)
                          }
                        }
                        n3241 = local read "SIG LAB02-2"() -> (w5883:T2)
                        n3242 = local read "SIG LAB02-1"() -> (w5885:T2)
                        n3243 = Bundle By Name(cluster=w5883, "Tmp Live"=w5861, "Tmp Neut"=w5860) -> (w5882:T2)
                        n3244 = Bundle By Name(cluster=w5885, "Tmp Live"=w5865, "Tmp Neut"=w5864) -> (w5884:T2)
                        n3245 = local write "SIG LAB02-1"(w5884) -> ()
                        n3246 = local write "SIG LAB02-2"(w5882) -> ()
                      }
                      frame #3 {
                        n3247 = case shown="False" w5915 {
                          tunnel: [w5946 w5947] -> w5931
                          tunnel: w5914 -> [_ w5947]
                          frame False {
                            n3248 = local read "CAL LAB03"() -> (w5946:T15)
                          }
                          frame True {
                          }
                        }
                        n3249 = local read "TEMP LA03"() -> (w5921:T10)
                        n3250 = local read "LAB03 TEMP"() -> (w5922:T13)
                        n3251 = call "sub vi - temperature delay v4.vi"("2-run"=w5903, "1-run"=w5904, "temp values IN"=w5921, "temp signals"=w5922) -> ("T2-N"=w5916:dbl, "T2-L"=w5917:dbl, "T1-N"=w5918:dbl, "T1-L"=w5919:dbl, "temp values OUT"=w5920:T47)  [unwired: 3 in]
